vi "Convert Fit Parameters (tau to-from sigma).vi"(8 "Error In":errorcluster, 9 "tau ->sigma (F)/sigma->tau (T)":bool, 10 "Fit Model":T1 caption="Model", 11 "All Parameters in":dbl[](array[numeric])) -> (0 "Error Out":errorcluster, 3 "All Parameters out":dbl[](array[numeric]))   [LabVIEW 2021, in "Fits.lvlib"]
doc: "The VI expects that bounfs for all parameters of the model are provided.\n\nThis VI assumes that the <B>Fit Parameter Constraints</B> involve tau, and returns values which involve sigma = sqrt(tau).\n\nRescales the constraints according to the Y normalization factor."
uses:
  Fits.lvlib
  Decay Convolution/Decay Model.ctl
  <vilib>/Utility/error.llb/Error Cluster From Error Code.vi
  <vilib>/ErrorRing/Error Ring.xnode
panel:
  # "returns sigma = sqrt(abs(tau))"
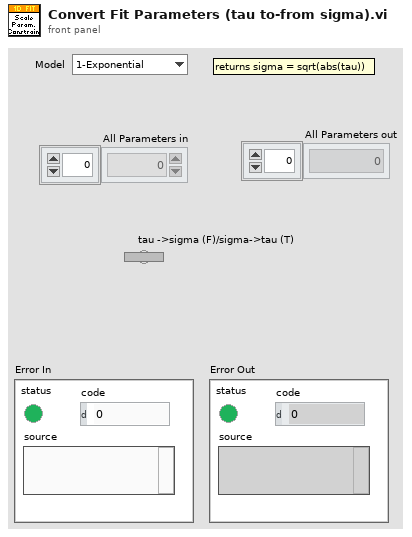
[diagram p1: front panel]
types:
  T1 = typedef "Fits.lvlib/Decay Model.ctl" = enum16{"1-Exponential", "2-Exponentials"}
  T2 = typedef "Fits.lvlib/Decay Fit Parameters In List.ctl" = enum16{"Offset", "Baseline", "A_1", "tau_1", "A_2", "tau_2"}
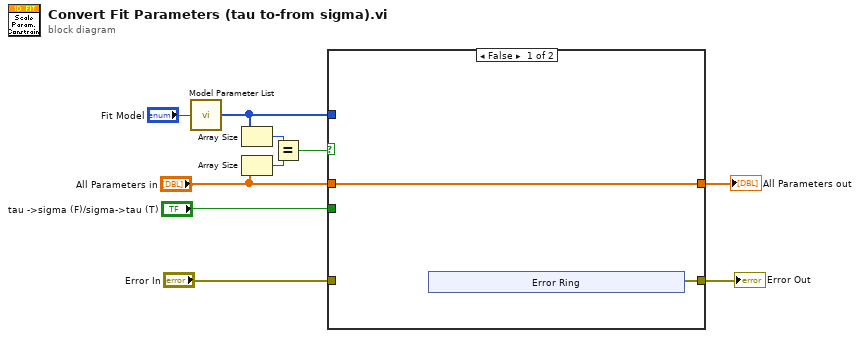
[diagram p0: block diagram]
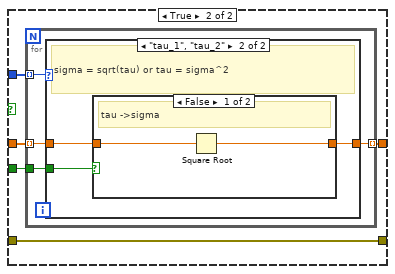
[diagram p2: hidden frame]
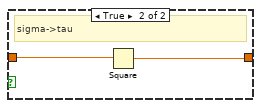
[diagram p4: hidden frame]
diagram:
  n1 = call "Model Parameter List.vi"("Fit Model"="Fit Model") -> ("Model Parameter List"=w9:T2[])
  n2 = Array Size(array=w9) -> (size(s)=w8:i32)
  n3 = Array Size(array="All Parameters in") -> (size(s)=w7:i32)
  n4 = Equal?(x=w8, y=w7) -> (x = y?=w3:bool)
  n5 = case shown="False" w3 {
    tunnel: w9 -> [_ w21]
    tunnel: "All Parameters in" -> [w11 w20]
    tunnel: "Error In" -> [_ w19]
    tunnel: [w12 w19] -> w5
    tunnel: [w11 w18] -> w2
    tunnel: "tau ->sigma (F)/sigma->tau (T)" -> [_ w17]
    frame False {
      n6 = xnode "Error Ring"() -> ("error out"=w12:errorcluster)
    }
    frame True {
      n7 = for {
        tunnel: w20 -> [w24] mode=indexing
        tunnel: w21 -> [w25] mode=indexing
        tunnel: [w23] -> w18 mode=indexing
        tunnel: w17 -> [w22]
        n8 = case shown="\"tau_1\", \"tau_2\"" w25 {
          tunnel: w24 -> [w26 w28]
          tunnel: [w26 w27] -> w23
          tunnel: w22 -> [_ w29]
          frame "Offset", Default {
            # "should have been set to some finite values"
          }
          frame "tau_1", "tau_2" {
            # "sigma = sqrt(tau) or tau = sigma^2"
            n9 = case shown="False" w29 {
              tunnel: w28 -> [w31 w33]
              tunnel: [w30 w32] -> w27
              frame False {
                # "tau ->sigma"
                n10 = Square Root(x=w31) -> (sqrt(x)=w30:dbl)
              }
              frame True {
                # "sigma->tau"
                n11 = Square(x=w33) -> (x^2=w32:dbl)
              }
            }
          }
        }
      }
    }
  }
  "Error Out" <- w5
  "All Parameters out" <- w2
